vi "Typecast Thermocouple.vi"(8 "error in (no error)":errorcluster, 10 "Thermocouple Type":string, 11 "Thermocouple in":refnum<class "Thermocouple.lvclass">) -> (0 "error out":errorcluster, 3 "Thermocouple out":refnum<class "Thermocouple.lvclass">)   [LabVIEW 2018, in "Thermocouple.lvlib" / "Thermocouple.lvclass"]
uses:
  Thermocouple.lvclass
  Custom Controls/Thermocouple Type.ctl
  Thermocouple.lvclass/Thermocouple.ctl
  Thermocouple.lvlib
panel:
  in  "Thermocouple Typedef":T1
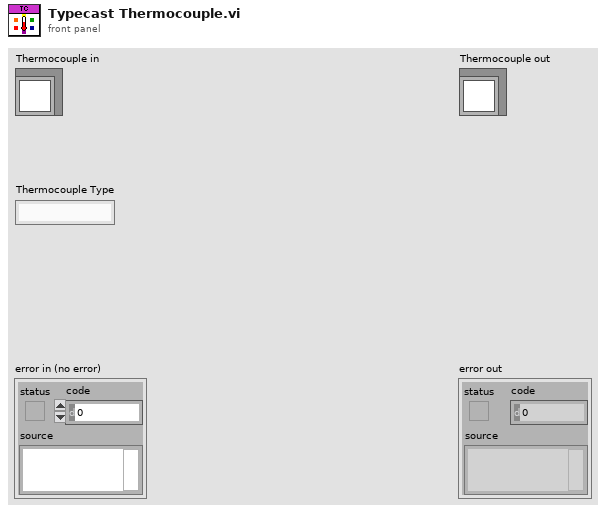
[diagram p1: front panel]
types:
  T1 = typedef "Thermocouple.lvlib/Thermocouple Type.ctl" = enum16{"J", "K", "N", "R", "S", "T", "B", "E"}
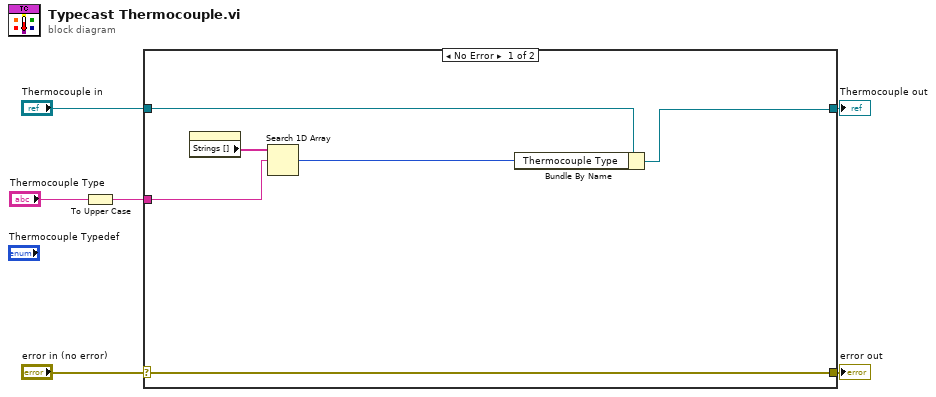
[diagram p0: block diagram]
diagram:
  n1 = To Upper Case(1:"Thermocouple Type") -> (0:w1:string)
  n2 = case shown="No Error" "error in (no error)" {
    selector: "error in (no error)" -> [w12 w14]
    tunnel: [w12 w14] -> w5
    tunnel: [w7 w13] -> w3
    tunnel: "Thermocouple in" -> [w11 w13]
    tunnel: w1 -> [w9 _]
    frame No Error {
      n3 = property on="Thermocouple Typedef" class="Enum (strict)"() -> ("Strings []"=w10:string[])  [unwired: 2 in, 2 out]
      n4 = Search 1D Array(1D array=w10, element=w9) -> (index of element=w8:i32)  [unwired: 1 in]
      n5 = Bundle By Name(cluster=w11, "Thermocouple Type"=w8) -> (w7:refnum<class "Thermocouple.lvclass">)
    }
    frame Error {
    }
  }
  "error out" <- w5
  "Thermocouple out" <- w3
